vi "tool_Unicode_Convert Unicode to ASCII (Scalar) Exaprom.vi"(4 "Unicode":string) -> (1 "ASCII":string)   [LabVIEW 2019]
uses:
  kernel32.dll
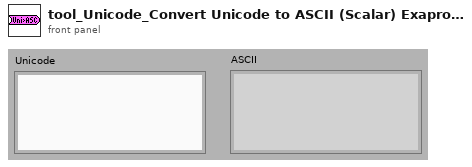
[diagram p1: front panel]
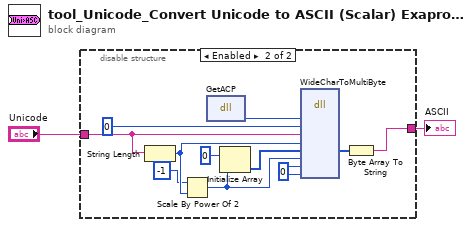
[diagram p0: block diagram]
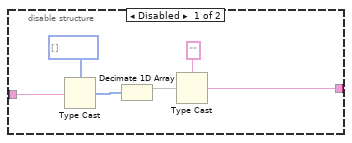
[diagram p2: hidden frame]
diagram:
  n1 = disable-structure shown="Enabled" {
    disable-tunnel: "Unicode" -> [w8 w14]
    disable-tunnel: [w5 w13] -> w1
    frame Disabled {
      n2 = Type Cast(type=u8[] [], x=w8) -> (*(type *) &x=w4:u8[])
      n3 = Decimate 1D Array(w4) -> (w3:u8[])  [unwired: 1 out]
      n4 = Type Cast(type="", x=w3) -> (*(type *) &x=w5:string)
    }
    frame Enabled {
      w9 = u32 0
      n5 = String Length(string=w14) -> (length=w12:i32)
      n6 = Scale By Power Of 2(n=-1, x=w12) -> (x*2^n=w10:i32)
      n7 = dll-call lib="kernel32.dll" fn="GetACP" label="GetACP()"() -> (w19:u32)  [unwired: 3 in, 2 out]
      n8 = Initialize Array(u8 0, w10) -> (w17:u8[])
      n9 = dll-call lib="kernel32.dll" fn="WideCharToMultiByte"("codePage"=w19, "dwFlags"=u32 0, "lpWideCharStr"=w14, "cchWideChar"=w12, "lpMultiByteStr"=w17, "cbMultiByte"=w10, "lpDefaultChar"=w9, "lpUsedDefaultChar"=w9) -> ("lpMultiByteStr"=w18:u8[])  [unwired: 10 in, 3 out]
      n10 = Byte Array To String(unsigned byte array=w18) -> (string=w13:string)
    }
  }
  "ASCII" <- w1
